vi "Resolution Check Popup.vi"(8 "error in":errorcluster, 11 "SR for Check":T1 {"Last Updated" format="%<%x>T"}) -> (0 "error out":errorcluster, 2 "Passed Off?":bool, 3 "Window Closed?":bool)   [LabVIEW 2018]
uses:
  SR Cluster.ctl
  SR Status.ctl
  <vilib>/Utility/miscctls.llb/LVPointTypeDef.ctl
  <vilib>/Utility/miscctls.llb/LVRectTypeDef.ctl
panel:
  in  "Resolved":bool
  in  "Passed Off":bool
  out "SR Information":string
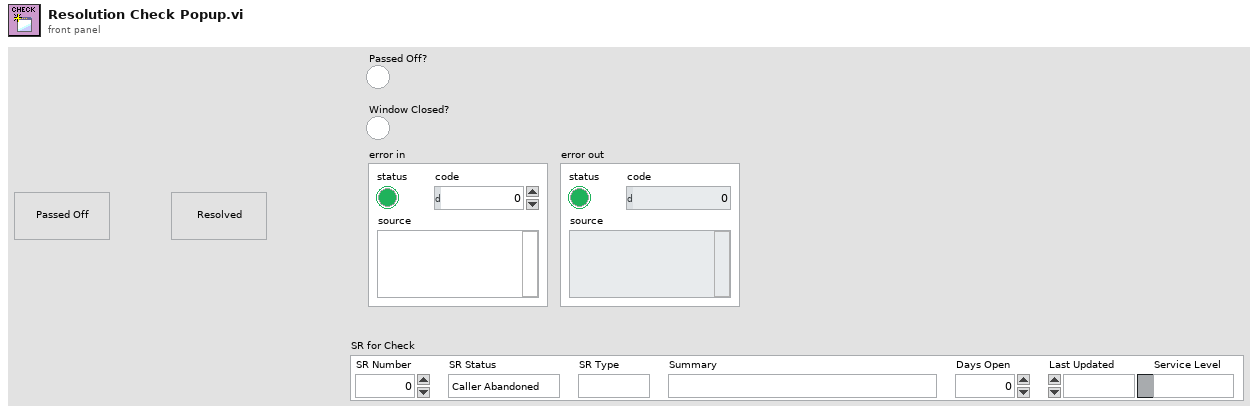
[diagram p1: front panel]
types:
  T1 = typedef "SR Cluster.ctl" = cluster{"SR Number":i32, "SR Type":string, "Summary":string, "Days Open":dbl, "Last Updated":timestamp, "Service Level":string, "SR Status":T2}
  T2 = typedef "SR Status.ctl" = enum16{"Caller Abandoned", "Created in Error", "Expired", "Forum Resolved AE", "Forum Resolved Customer", "IN WORK", "IN WORK Collab with AES", "IN WORK Collab with PSE", "IN WORK Collab with SE", "IN WORK Customer Added Note", "IN WORK Escalation", "IN WORK Wait on Customer", "Open", "Potentially Resolved", "Presumed Resolved", "RMA Approved for Return", "Resolved", "Passed Off"}
  T3 = typedef "LVRectTypeDef.ctl" = cluster{"Left":i16, "Top":i16, "Right":i16, "Bottom":i16}
  T4 = typedef "LVPointTypeDef.ctl" = cluster{"Horizontal":i16, "Vertical":i16}
  T5 = typedef "LVBoundsTypeDef.ctl" = cluster{"Width":u32, "Height":u32}
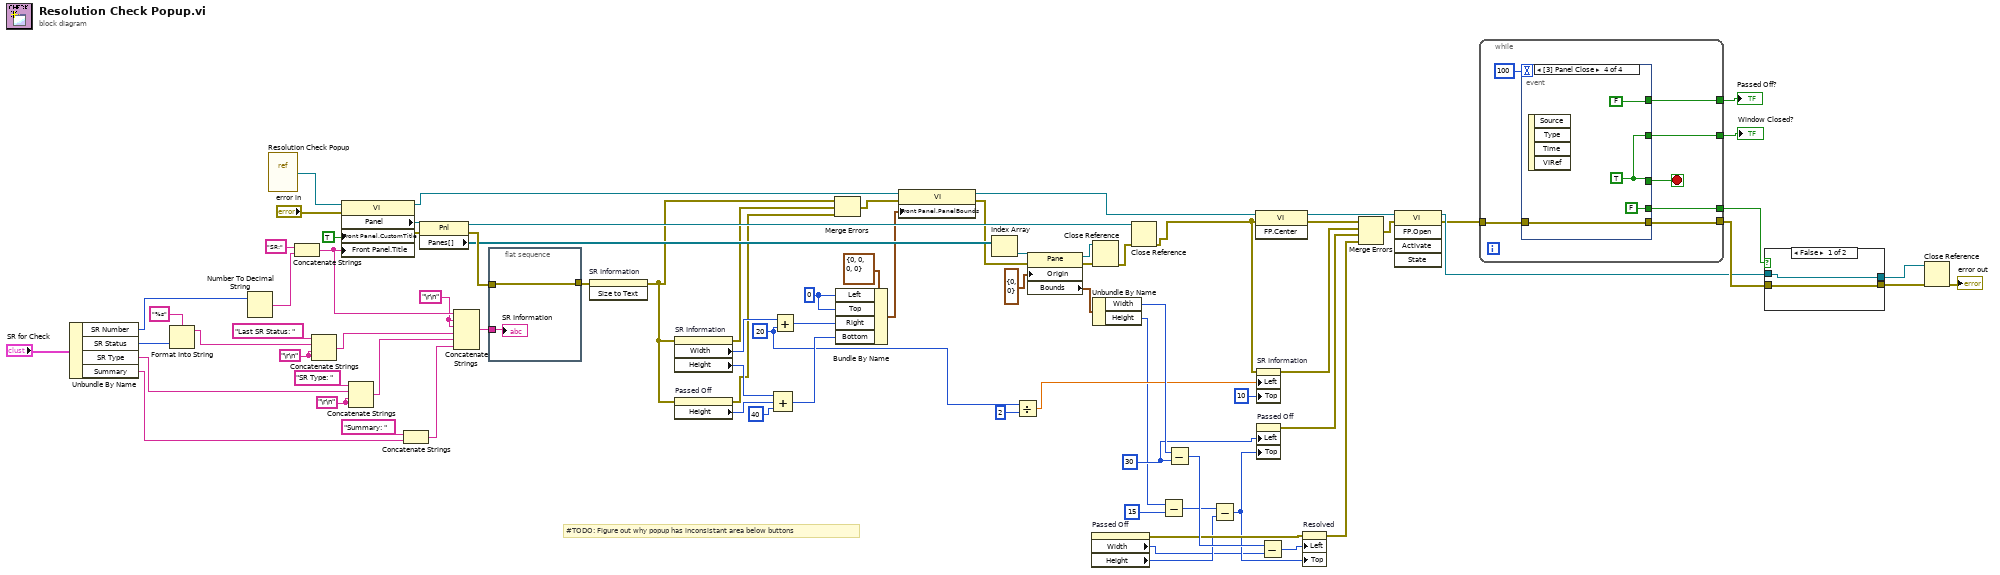
[diagram p0: block diagram]
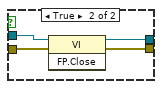
[diagram p2: hidden frame]
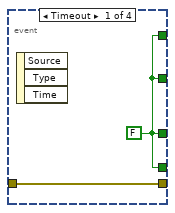
[diagram p3: hidden frame]
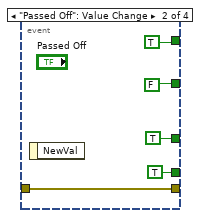
[diagram p4: hidden frame]
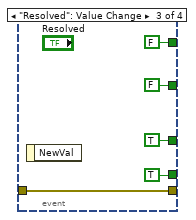
[diagram p5: hidden frame]
diagram:
  w33 = 30 ("Position:Left")
  w32 = u32 20 ("y")
  w44 = i16 0 ("Left")
  w29 = "\r\n"
  w28 = "\r\n"
  w25 = "\r\n"
  # "#TODO: Figure out why popup has inconsistant area below buttons"
  n1 = Unbundle By Name("SR for Check") -> ("SR Number"=w57:i32, "SR Status"=w9:T2, "SR Type"=w50:string, "Summary"=w51:string)
  n2 = Format Into String(format string="%s", w9) -> (resulting string=w7:string)  [unwired: 2 in, 1 out]
  n3 = Number To Decimal String(number=w57) -> (decimal integer string=w61:string)  [unwired: 1 in]
  n4 = vi-ref "Resolution Check Popup.vi"() -> (w74:refnum<vi>)
  n5 = Concatenate Strings("SR:" ("string"), w61) -> (w56:string)
  n6 = Concatenate Strings("Last SR Status: " ("string"), w7, w28, w28) -> (w27:string)
  n7 = property class="VI"(reference=w74, error in="error in", "Front Panel.CustomTitle"=TRUE ("Front Panel Window:Custom Title"), "Front Panel.Title"=w56) -> (reference out=w49:refnum<vi>, error out=w75:errorcluster, "Panel"=w76:refnum<vi>)
  n8 = Concatenate Strings("SR Type: " ("string"), w50, w29, w29) -> (w26:string)
  n9 = Concatenate Strings("Summary: " ("string"), w51) -> (w24:string)
  n10 = property class="Pnl"(reference=w76, error in=w75) -> (reference out=w77:refnum<vi>, error out=w60:errorcluster, "Panes[]"=w59:refnum<vi>[])
  n11 = Concatenate Strings(w56, w25, w25, w27, w26, w24) -> (w55:string)
  n12 = flat-sequence {
    tunnel: [w84] -> w11
    tunnel: w60 -> [w84]
    tunnel: w55 -> [w83]
    frame #0 {
      "SR Information" <- w83
    }
  }
  n13 = invoke on="SR Information" class="Str" method="Size to Text"(error in=w11) -> (error out=w5:errorcluster)  [unwired: 2 in, 2 out]
  n14 = property on="SR Information" class="Str"(error in=w5) -> (error out=w4:errorcluster, "Width"=w12:u32, "Height"=w13:u32)  [unwired: 1 in, 1 out]
  n15 = property on="Passed Off" class="Bool"(error in=w5) -> (error out=w3:errorcluster, "Height"=w41:u32)  [unwired: 1 in, 1 out]
  n16 = Add(x=w12, y=w32) -> (x+y=w42:u32)
  n17 = Compound Arithmetic op=ADD(w13, w41, u32 40 ("y")) -> (w43:u32)
  n18 = Merge Errors(w5, w4, w3) -> (w2:errorcluster)
  n19 = Bundle By Name(cluster=T3 {"Left"=0, "Top"=0, "Right"=0, "Bottom"=0} ("Front Panel Window:Panel Bounds"), "Left"=w44, "Top"=w44, "Right"=w42, "Bottom"=w43) -> (w45:T3)
  n20 = property class="VI"(reference=w49, error in=w2, "Front Panel.PanelBounds"=w45) -> (reference out=w47:refnum<vi>, error out=w48:errorcluster)
  n21 = Index Array(array=w59) -> (element=w82:refnum<vi>)  [unwired: 1 in]
  n22 = Divide(x=w32, y=u32 2) -> (x/y=w30:dbl)
  n23 = property class="Pane"(reference=w82, error in=w48, "Origin"=T4 {"Horizontal"=0, "Vertical"=0}) -> (reference out=w80:refnum<vi>, error out=w79:errorcluster, "Bounds"=w63:T5)
  n24 = property on="Passed Off" class="Bool"() -> (error out=w20:errorcluster, "Width"=w15:u32, "Height"=w16:u32)  [unwired: 2 in, 1 out]
  n25 = Close Reference(reference=w80, error in (no error)=w79) -> (error out=w78:errorcluster)
  n26 = Unbundle By Name(w63) -> ("Width"=w40:u32, "Height"=w19:u32)
  n27 = Close Reference(reference=w77, error in (no error)=w78) -> (error out=w1:errorcluster)
  n28 = Subtract(x=w19, y=u32 15) -> (x-y=w18:u32)
  n29 = Subtract(x=w40, y=w33) -> (x-y=w39:u32)
  n30 = Subtract(x=w18, y=w16) -> (x-y=w17:u32)
  n31 = invoke class="VI" method="FP.Center"(reference=w47, error in=w1) -> (reference out=w66:refnum<vi>, error out=w38:errorcluster)  [unwired: 1 in, 1 out]
  n32 = property on="SR Information" class="Str"(error in=w1, "Left"=w30, "Top"=10 ("Position:Top")) -> (error out=w36:errorcluster)  [unwired: 1 in, 1 out]
  n33 = property on="Passed Off" class="Bool"("Left"=w33, "Top"=w17) -> (error out=w35:errorcluster)  [unwired: 2 in, 1 out]
  n34 = Subtract(x=w39, y=w15) -> (x-y=w21:u32)
  n35 = property on="Resolved" class="Bool"(error in=w20, "Left"=w21, "Top"=w17) -> (error out=w34:errorcluster)  [unwired: 1 in, 1 out]
  n36 = Merge Errors(w38, w36, w35, w34) -> (w37:errorcluster)
  n37 = invoke class="VI" method="FP.Open"(reference=w66, error in=w37) -> (reference out=w68:refnum<vi>, error out=w67:errorcluster)  [unwired: 3 in, 3 out]
  n38 = while {
    tunnel: w67 -> [w90]
    tunnel: [w91] -> w72
    tunnel: [w87] -> w65
    tunnel: [w86] -> w64
    tunnel: [w85] -> w6
    stop <- w88 stop-if-true
    n39 = event shown="[3] Panel Close" {
      selector: _ -> [_ _ _ _]
      dyn-events: _ -> [_ _ _ _]
      timeout: 100 -> [_ _ _ _]
      tunnel: [w93 w95 w100 w105] -> w91
      tunnel: w90 -> [w93 w95 w100 w105]
      tunnel: [w92 TRUE TRUE w107] -> w88
      tunnel: [w92 FALSE FALSE w107] -> w87
      tunnel: [w92 TRUE FALSE FALSE] -> w86
      tunnel: [w92 TRUE TRUE FALSE] -> w85
      event Timeout {
        w92 = FALSE
        n40 = event-data() -> ()  [unwired: 1 in, 3 out]
      }
      event "Passed Off": Value Change {
        n41 = event-data() -> ()  [unwired: 1 in, 1 out]
      }
      event "Resolved": Value Change {
        n42 = event-data() -> ()  [unwired: 1 in, 1 out]
      }
      event Panel Close {
        w107 = TRUE
        n43 = event-data() -> ()  [unwired: 1 in, 4 out]
      }
    }
  }
  "Passed Off?" <- w64
  "Window Closed?" <- w65
  n44 = case shown="False" w6 {
    tunnel: [w108 w113] -> w73
    tunnel: w72 -> [w108 w112]
    tunnel: w68 -> [w109 w111]
    tunnel: [w109 w110] -> w10
    frame False {
    }
    frame True {
      n45 = invoke class="VI" method="FP.Close"(reference=w111, error in=w112) -> (reference out=w110:refnum<vi>, error out=w113:errorcluster)  [unwired: 1 in, 1 out]
    }
  }
  n46 = Close Reference(reference=w10, error in (no error)=w73) -> (error out=→"error out":errorcluster)
